vi "User_Change.vi"() -> ()   [LabVIEW 2020]
panel:
  in  "User_Password":string caption="密        码"
  in  "Ok":bool
  in  "User_Name":string caption="用  户  名"
  # "切换用户"
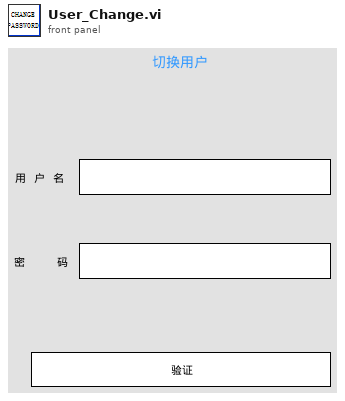
[diagram p1: front panel]
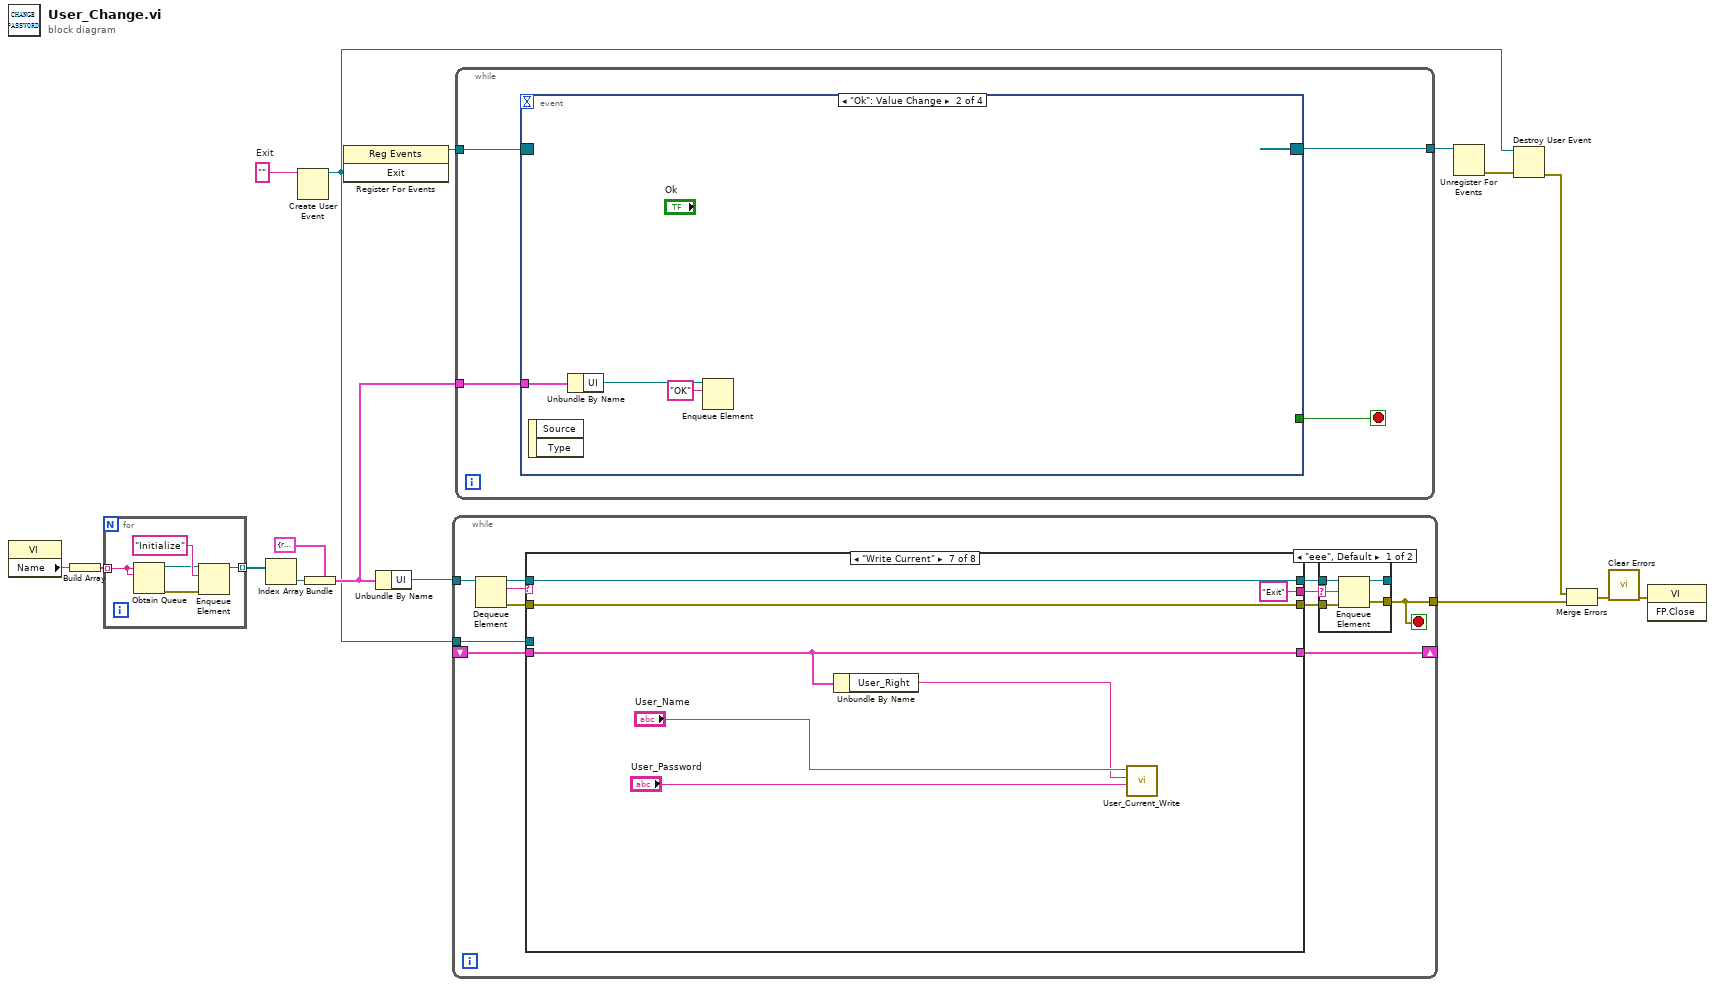
[diagram p0: block diagram]
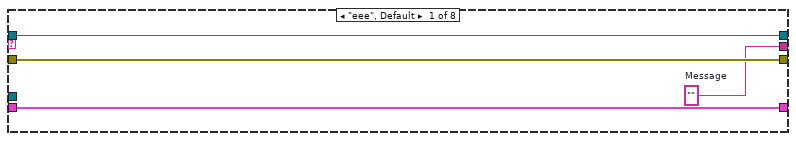
[diagram p3: hidden frame]
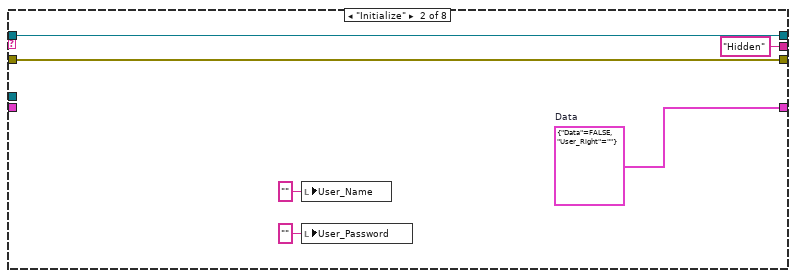
[diagram p4: hidden frame]
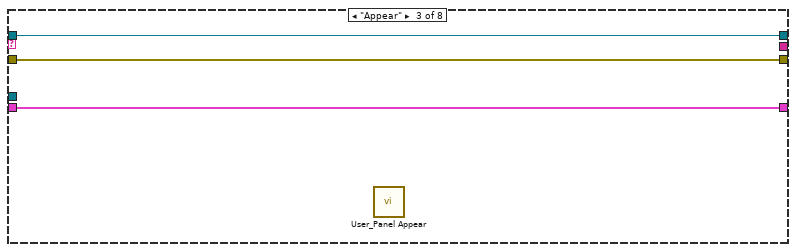
[diagram p5: hidden frame]
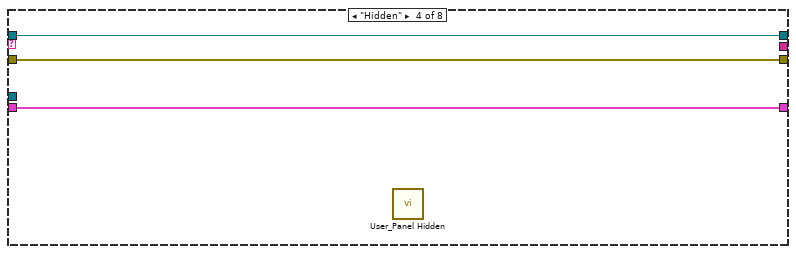
[diagram p6: hidden frame]
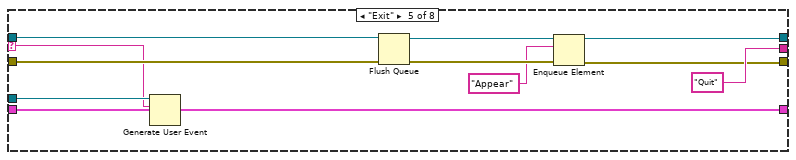
[diagram p7: hidden frame]
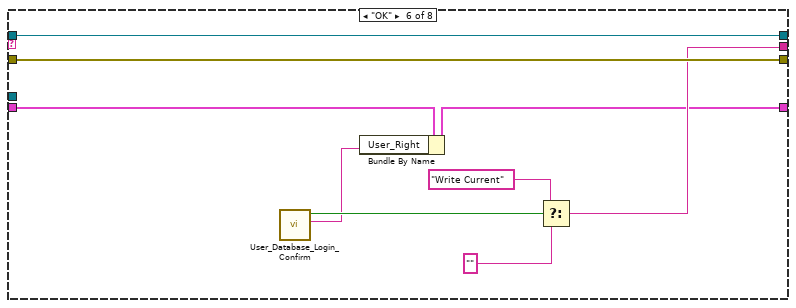
[diagram p8: hidden frame]
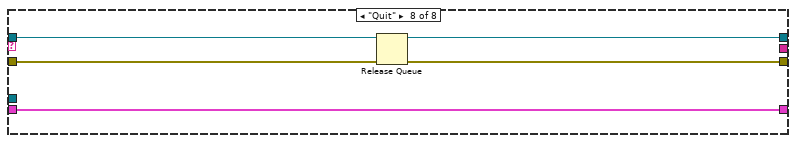
[diagram p9: hidden frame]
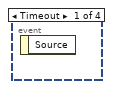
[diagram p10: hidden frame]
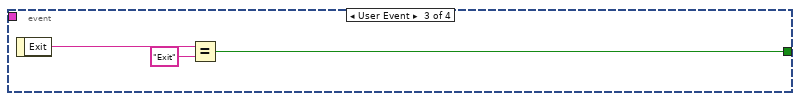
[diagram p11: hidden frame]
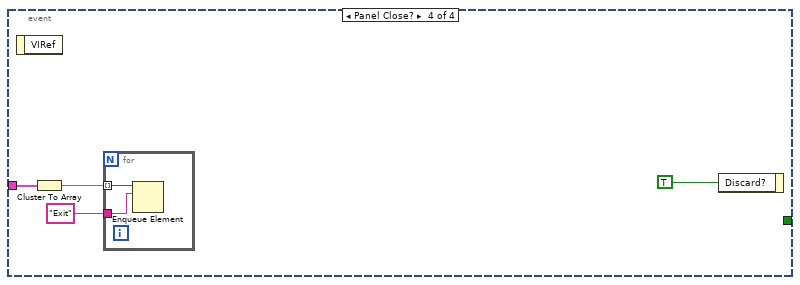
[diagram p12: hidden frame]
diagram:
  w2 = ""  # Exit
  n1 = property class="VI"() -> ("Name"=w12:string)  [unwired: 2 in, 2 out]
  n2 = Build Array(w12) -> (w13:string[])
  n3 = for {
    tunnel: w13 -> [w17] mode=indexing
    tunnel: [w18] -> w7 mode=indexing
    n4 = Obtain Queue(name (unnamed)=w17, element data type=w17) -> (queue out=w20:refnum<queue>, error out=w19:errorcluster)  [unwired: 3 in, 1 out]
    n5 = Enqueue Element(queue=w20, element="Initialize" ("元素"), error in (no error)=w19) -> (queue out=w18:refnum<queue>)  [unwired: 1 in, 2 out]
  }
  n6 = Index Array(array=w7) -> (element=w10:refnum<queue>)  [unwired: 1 in]
  n7 = Create User Event(user event datatype=w2) -> (user event=w6:refnum<user-event>)  [unwired: 1 in, 1 out]
  n8 = Bundle(cluster=cluster{"UI":refnum<queue>} {"UI"=refnum}, "UI"=w10) -> (w11:cluster{"UI":refnum<queue>})
  n9 = register-events(w6) -> (reference out=w3:refnum<event-registration>)  [unwired: 2 in, 1 out]
  n10 = Unbundle By Name(w11) -> ("UI"=w8:refnum<queue>)
  n11 = while {
    tunnel: w8 -> [w32]
    tunnel: [w22] -> w15
    shift-right: [w26] -> _
    shift-left: _ -> [w25]
    tunnel: w6 -> [w24]
    stop <- w22 stop-if-true
    n12 = Dequeue Element(queue=w32) -> (queue out=w31:refnum<queue>, element=w23:string, error out=w28:errorcluster)  [unwired: 2 in, 1 out]
    n13 = case shown="\"Write Current\"" w23 {
      selector: w23 -> [_ _ _ _ w61 _ _ _]
      tunnel: w31 -> [w43 w49 w52 w55 w64 w75 w82 w86]
      tunnel: [w43 w49 w52 w55 w57 w75 w82 w86] -> w30
      tunnel: [w42 w48 w51 w54 w58 w74 w81 w83] -> w29
      tunnel: w28 -> [w42 w48 w51 w54 w63 w74 w81 w85]
      tunnel: [w41 "Hidden" ("Message") _ _ "Quit" ("Message") w69 "Exit" ("Message") _] -> w27
      tunnel: [w40 w47 w50 w53 w66 w68 w77 w84] -> w26
      tunnel: w25 -> [w40 _ w50 w53 w66 w73 w77 w84]
      tunnel: w24 -> [_ _ _ _ w62 _ _ _]
      frame "eee", Default {
        w41 = ""  # Message
      }
      frame "Initialize" {
        w47 = cluster{"Data":bool, "User_Right":string} {"Data"=FALSE, "User_Right"=""}  # Data
        n14 = local write "User_Name"("" ("User_Name")) -> ()
        n15 = local write "User_Password"("" ("User_Password")) -> ()
      }
      frame "Appear" {
        n16 = call "User_Panel Appear.vi"() -> ()  [unwired: 11 in, 1 out]
      }
      frame "Hidden" {
        n17 = call "User_Panel Hidden.vi"() -> ()  [unwired: 11 in, 1 out]
      }
      frame "Exit" {
        n18 = Generate User Event(user event=w62, event data cluster=w61) -> ()  [unwired: 2 in, 2 out]
        n19 = Flush Queue(queue=w64, error in (no error)=w63) -> (queue out=w60:refnum<queue>, error out=w59:errorcluster)  [unwired: 1 out]
        n20 = Enqueue Element(queue=w60, element="Appear" ("Message"), error in (no error)=w59) -> (queue out=w57:refnum<queue>, error out=w58:errorcluster)  [unwired: 1 in, 1 out]
      }
      frame "OK" {
        n21 = call "User_Database_Login_Confirm.vi"() -> ("User_Right"=w67:string, "OK"=w70:bool)  [unwired: 9 in, 1 out]
        n22 = Bundle By Name(cluster=w73, "User_Right"=w67) -> (w68:cluster{"Data":bool, "User_Right":string})
        n23 = Select(t="Write Current", s=w70, f="") -> (s? t:f=w69:string)
      }
      frame "Write Current" {
        n24 = Unbundle By Name(w77) -> ("User_Right"=w76:string)
        n25 = call "User_Current_Write.vi"("Password"="User_Password", "User_Right"=w76, "Name"="User_Name") -> ()  [unwired: 8 in, 1 out]
      }
      frame "Quit" {
        n26 = Release Queue(queue=w86, error in (no error)=w85) -> (error out=w83:errorcluster)  [unwired: 1 in, 2 out]
      }
    }
    n27 = case shown="\"eee\", Default" w27 {
      selector: w27 -> [w33 _]
      tunnel: w30 -> [w37 w39]
      tunnel: w29 -> [w36 w38]
      tunnel: [w35 w38] -> w22
      tunnel: [w34 w39] -> _
      frame "eee", Default {
        n28 = Enqueue Element(queue=w37, element=w33, error in (no error)=w36) -> (queue out=w34:refnum<queue>, error out=w35:errorcluster)  [unwired: 1 in, 1 out]
      }
      frame "" {
      }
    }
  }
  n29 = while {
    tunnel: w3 -> [w89]
    tunnel: [w88] -> w5
    tunnel: w11 -> [w87]
    stop <- w90 stop-if-true
    n30 = event shown="[1] \"Ok\": Value Change" {
      selector: w89 -> [_ _ _ _]
      dyn-events: [_ _ _ _] -> w88
      timeout: _ -> [_ _ _ _]
      tunnel: [_ _ w95 _] -> w90
      tunnel: w87 -> [_ w93 _ w99]
      event Timeout {
        n31 = event-data() -> ()  [unwired: 1 in, 1 out]
      }
      event "Ok": Value Change {
        n32 = event-data() -> ()  [unwired: 1 in, 2 out]
        n33 = Unbundle By Name(w93) -> ("UI"=w92:refnum<queue>)
        n34 = Enqueue Element(queue=w92, element="OK" ("元素")) -> ()  [unwired: 2 in, 3 out]
      }
      event User Event {
        n35 = event-data() -> ("Exit"=w96:string)  [unwired: 1 in]
        n36 = Equal?(x=w96, y="Exit") -> (x = y?=w95:bool)
      }
      event Panel Close? {
        n37 = event-data() -> ()  [unwired: 1 in, 1 out]
        n38 = Cluster To Array(cluster=w99) -> (array=w98:refnum<queue>[])
        n39 = for {
          tunnel: w98 -> [w102] mode=indexing
          tunnel: "Exit" ("元素") -> [w101]
          n40 = Enqueue Element(queue=w102, element=w101) -> ()  [unwired: 2 in, 3 out]
        }
        n41 = event-data("Discard?"=TRUE ("放弃？")) -> ()  [unwired: 1 in, 1 out]
      }
    }
  }
  n42 = Unregister For Events(event registration refnum=w5) -> (error out=w4:errorcluster)  [unwired: 1 in]
  n43 = Destroy User Event(user event=w6, error in=w4) -> (error out=w14:errorcluster)
  n44 = Merge Errors(w14, w15) -> (w16:errorcluster)
  n45 = call <vilib>:"Clear Errors.vi"("error in (no error)"=w16) -> ("error out"=w1:errorcluster)  [unwired: 5 in, 1 out]
  n46 = invoke class="VI" method="FP.Close"(error in=w1) -> ()  [unwired: 2 in, 3 out]
